vi "dilutionCalcR2.vi"(0 "Clust Refnum":refnum<vi>) -> ()   [LabVIEW 2011]
uses:
  source_dilution.ctl
  source_noDilution.ctl
panel:
  in  "Ga bubbler":T1={"Dilution"=FALSE, "Calculated"=0, "MFC1 flow"=0.0, "MFC2 flow"=10.0, "MFC3 flow"=100.0, "Main"={"Flow"=0.0, "Prep"=FALSE, "Run"=FALSE, "Active"=FALSE, "Name"=""}} caption="Al" {"Main"."Flow" format="%.2f"; "MFC1 flow" format="%.4f"; "MFC3 flow" format="%.1f"; "MFC2 flow" format="%.2f"; "Calculated" items=["Flow", "MFC1", "MFC2", "MFC3"]}
  in  "Al bubbler":T2 caption="Al" {"Flow" format="%.2f"}
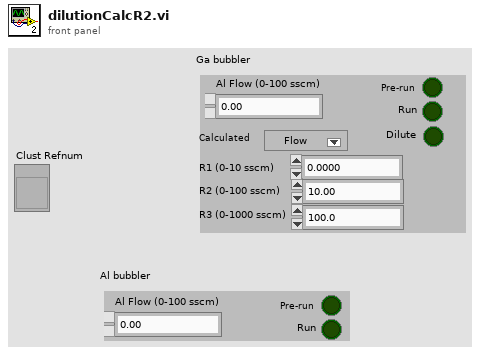
[diagram p1: front panel]
types:
  T1 = typedef "source_dilution.ctl" = cluster{"Dilution":bool, "Calculated":u16, "MFC1 flow":dbl, "MFC2 flow":dbl, "MFC3 flow":dbl, "Main":T2}
  T2 = typedef "source_noDilution.ctl" = cluster{"Flow":dbl, "Prep":bool, "Run":bool, "Active":bool, "Name":string}
  T3 = enum8{"Enabled", "Disabled", "Disabled and Grayed Out"}
  T4 = cluster{"Controls[][0]":refnum<vi>, "Controls[][1]":refnum<vi>, "Controls[][2]":refnum<vi>, "Controls[][3]":refnum<vi>, "Controls[][4]":refnum<vi>, "Controls[][5]":refnum<vi>, "Controls[][6]":refnum<vi>, "Controls[][7]":refnum<vi>, "Controls[][8]":refnum<vi>}
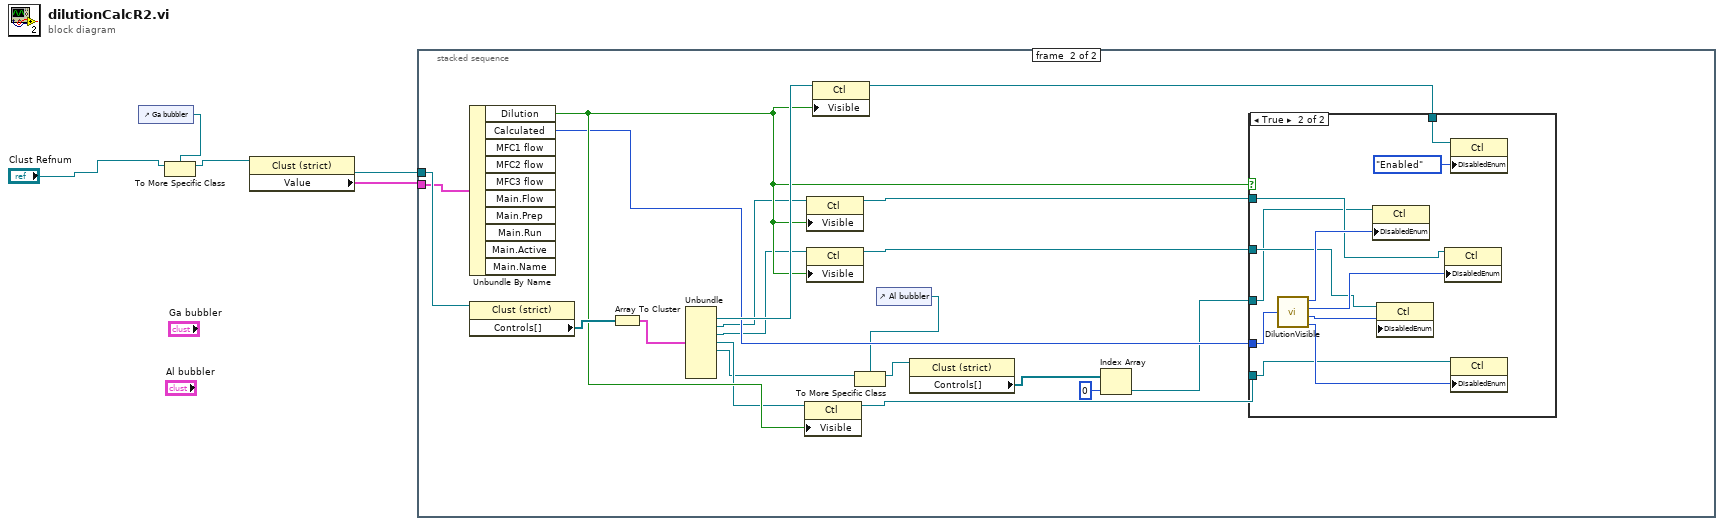
[diagram p0: block diagram]
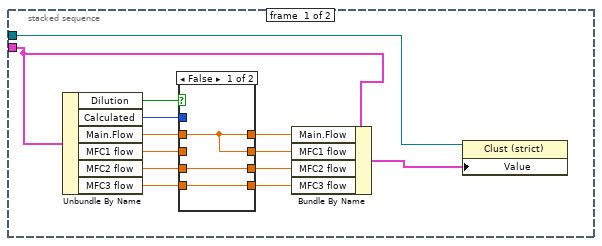
[diagram p2: hidden frame]
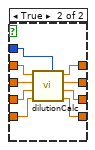
[diagram p3: hidden frame]
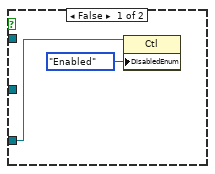
[diagram p4: hidden frame]
diagram:
  n1 = control-ref of="Ga bubbler"() -> (w3:refnum<vi>)
  n2 = To More Specific Class(target class=w3, reference="Clust Refnum") -> (specific class reference=w2:refnum<vi>)  [unwired: 1 in, 1 out]
  n3 = property on="Property Node" class="Clust (strict)"(reference=w2) -> (reference out=w5:refnum<vi>, "Value"=w4:T1)  [unwired: 1 in, 1 out]
  n4 = stacked-sequence {
    tunnel: w5 -> [w6 w50]
    tunnel: w4 -> [w8 w42]
    frame #0 {
      n5 = Unbundle By Name(w8) -> ("Dilution"=w18:bool, "Calculated"=w17:u16, "Main.Flow"=w14:dbl, "MFC1 flow"=w15:dbl, "MFC2 flow"=w16:dbl, "MFC3 flow"=w13:dbl)
      n6 = case shown="False" w18 {
        tunnel: w17 -> [_ w30]
        tunnel: w16 -> [w21 w27]
        tunnel: w15 -> [_ w28]
        tunnel: w14 -> [w19 w29]
        tunnel: w13 -> [w20 w26]
        tunnel: [w19 w25] -> w12
        tunnel: [w19 w24] -> w11
        tunnel: [w21 w23] -> w10
        tunnel: [w20 w22] -> w9
        frame False {
        }
        frame True {
          n7 = call "dilutionCalc.vi"("Calculated"=w30, "MFC3"=w26, "MFC2"=w27, "MFC1"=w28, "flow"=w29) -> ("MFC3 out"=w22:dbl, "MFC2 out"=w23:dbl, "MFC1 out"=w24:dbl, "flow out"=w25:dbl)  [unwired: 1 in]
        }
      }
      n8 = Bundle By Name(cluster=w8, "Main.Flow"=w12, "MFC1 flow"=w11, "MFC2 flow"=w10, "MFC3 flow"=w9) -> (w7:T1)
      n9 = property class="Clust (strict)"(reference=w6, "Value"=w7) -> ()  [unwired: 1 in, 2 out]
    }
    frame #1 {
      n10 = Unbundle By Name(w42) -> ("Dilution"=w46:bool, "Calculated"=w45:u16)  [unwired: 8 out]
      n11 = property class="Clust (strict)"(reference=w50) -> ("Controls[]"=w49:refnum<vi>[])  [unwired: 1 in, 2 out]
      n12 = Array To Cluster(array=w49) -> (cluster=w48:T4)
      n13 = Unbundle(w48) -> ("Controls[][1]"=w47:refnum<vi>, "Controls[][2]"=w41:refnum<vi>, "Controls[][3]"=w40:refnum<vi>, "Controls[][4]"=w39:refnum<vi>, "Controls[][5]"=w36:refnum<vi>)  [unwired: 4 out]
      n14 = property class="Ctl"(reference=w39, "Visible"=w46) -> (reference out=w38:refnum<vi>)  [unwired: 1 in, 1 out]
      n15 = property class="Ctl"(reference=w41, "Visible"=w46) -> (reference out=w43:refnum<vi>)  [unwired: 1 in, 1 out]
      n16 = property class="Ctl"(reference=w40, "Visible"=w46) -> (reference out=w44:refnum<vi>)  [unwired: 1 in, 1 out]
      n17 = property class="Ctl"(reference=w47, "Visible"=w46) -> (reference out=w37:refnum<vi>)  [unwired: 1 in, 1 out]
      n18 = control-ref of="Al bubbler"() -> (w31:refnum<vi>)
      n19 = To More Specific Class(target class=w31, reference=w36) -> (specific class reference=w35:refnum<vi>)  [unwired: 1 in, 1 out]
      n20 = property class="Clust (strict)"(reference=w35) -> ("Controls[]"=w34:refnum<vi>[])  [unwired: 1 in, 2 out]
      n21 = Index Array(array=w34, index=0) -> (element=w32:refnum<vi>)
      n22 = case shown="True" w46 {
        tunnel: w45 -> [_ w63]
        tunnel: w32 -> [w52 w55]
        tunnel: w44 -> [_ w57]
        tunnel: w43 -> [_ w56]
        tunnel: w38 -> [_ w58]
        tunnel: w37 -> [_ w54]
        frame False {
          n23 = property class="Ctl"(reference=w52, "DisabledEnum"=T3."Enabled" ("Disabled")) -> ()  [unwired: 1 in, 2 out]
        }
        frame True {
          n24 = call "DilutionVisible.vi"("calculated"=w63) -> ("flow"=w62:u16, "MFC1"=w61:u16, "MFC2"=w60:u16, "MFC3"=w59:u16)
          n25 = property class="Ctl"(reference=w55, "DisabledEnum"=w62) -> ()  [unwired: 1 in, 2 out]
          n26 = property class="Ctl"(reference=w57, "DisabledEnum"=w60) -> ()  [unwired: 1 in, 2 out]
          n27 = property class="Ctl"(reference=w56, "DisabledEnum"=w61) -> ()  [unwired: 1 in, 2 out]
          n28 = property class="Ctl"(reference=w54, "DisabledEnum"=T3."Enabled" ("Disabled")) -> ()  [unwired: 1 in, 2 out]
          n29 = property class="Ctl"(reference=w58, "DisabledEnum"=w59) -> ()  [unwired: 1 in, 2 out]
        }
      }
    }
  }
